vi "SQL_在指定表中修改列.vi"(8 "error in (no error)":errorcluster caption="错误输入（无错误）", 9 "字段类型":string="varchar(255)", 10 "字段名":string="d7", 11 "表名":string="test") -> (0 "error out":errorcluster caption="错误输出", 3 "SQL_在指定表中修改列":string)   [LabVIEW 2014]
doc: "该模板用于创建子VI。"
panel:
  # "varchar括号中的数值最大255"
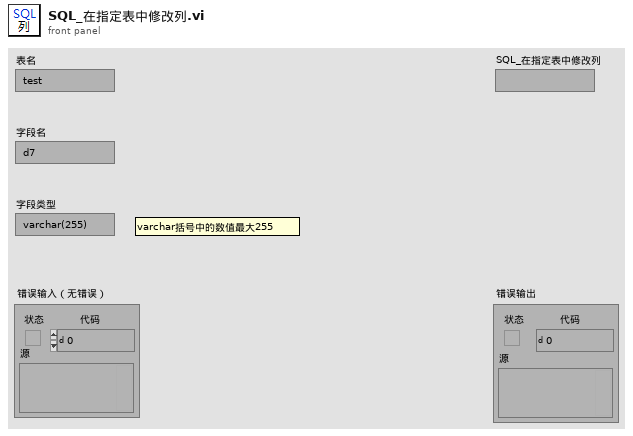
[diagram p1: front panel]
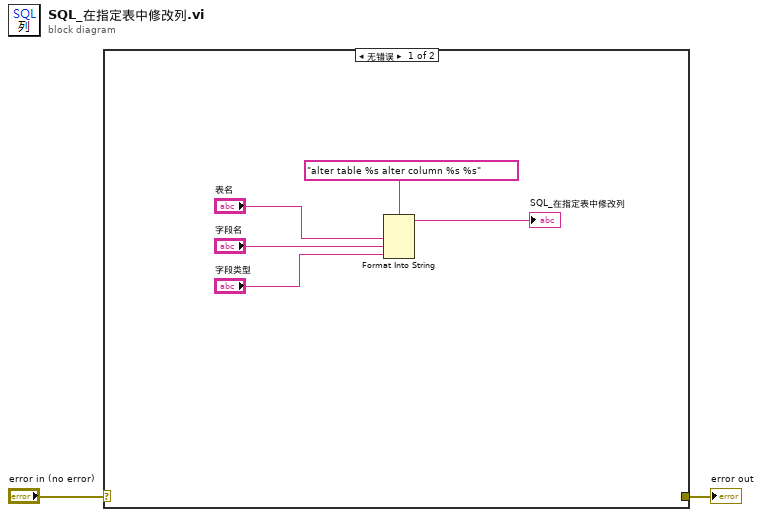
[diagram p0: block diagram]
diagram:
  n1 = case shown="无错误" "error in (no error)" {
    selector: "error in (no error)" -> [_ w8]
    tunnel: [_ w8] -> w1
    frame No Error {
      n2 = Format Into String(format string="alter table %s alter column %s %s", "表名", "字段名", "字段类型") -> (resulting string=→"SQL_在指定表中修改列":string)  [unwired: 2 in, 1 out]
    }
    frame Error {
    }
  }
  "error out" <- w1
